vi "FYP_VI_MIDI_KeyScanDataConvert.vi"(1 "KeyScan":i16) -> (0 "MIDI Note Number":i16)   [LabVIEW 2013]
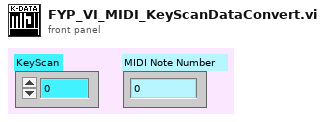
[diagram p1: front panel]
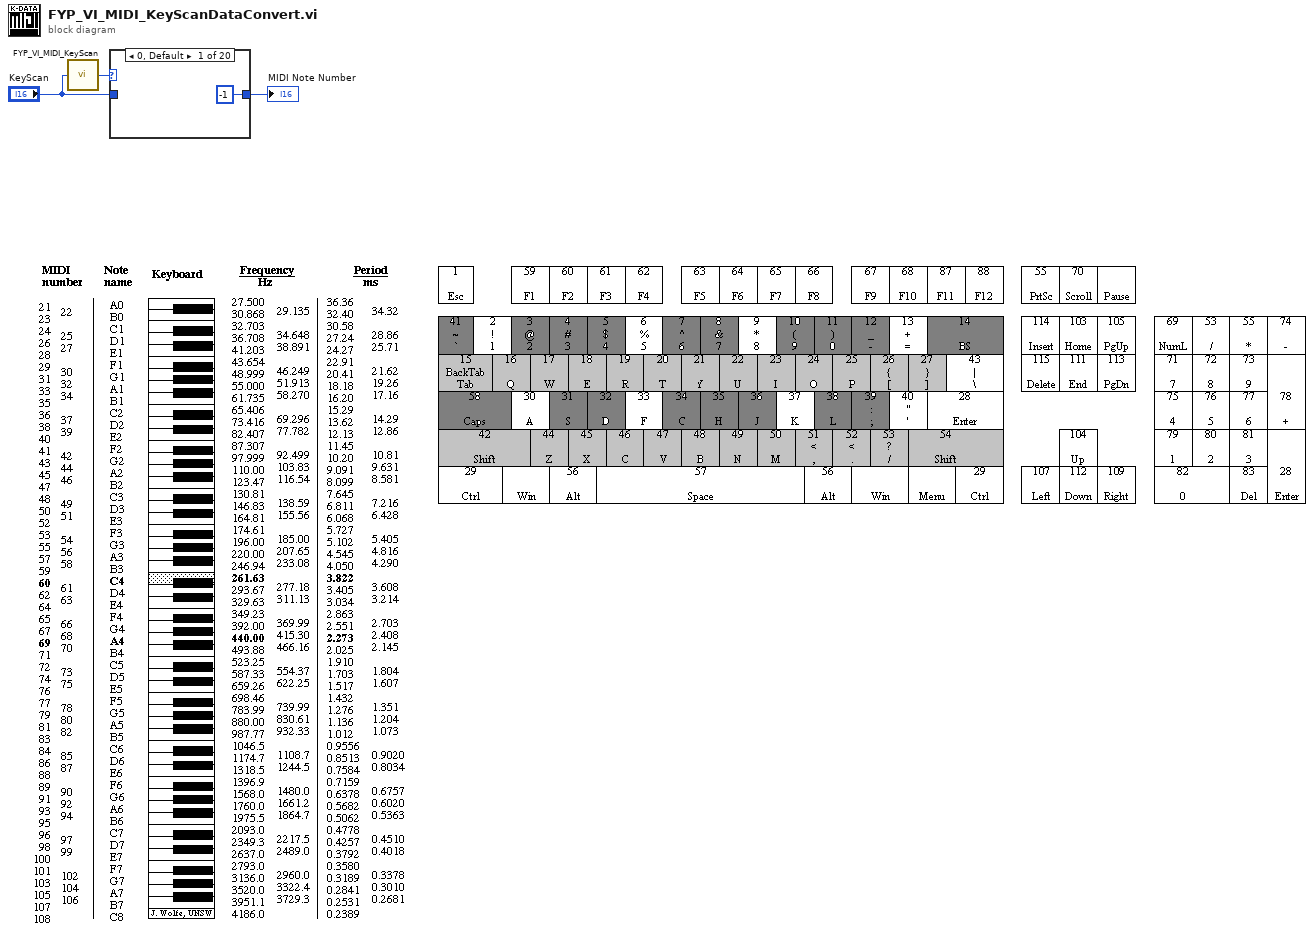
[diagram p0: block diagram]
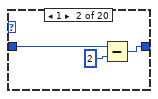
[diagram p2: hidden frame]
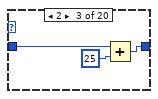
[diagram p3: hidden frame]
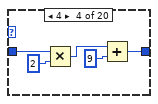
[diagram p4: hidden frame]
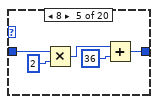
[diagram p5: hidden frame]
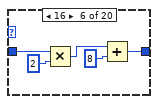
[diagram p6: hidden frame]
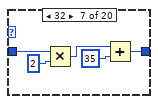
[diagram p7: hidden frame]
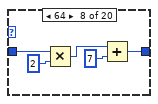
[diagram p8: hidden frame]
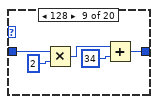
[diagram p9: hidden frame]
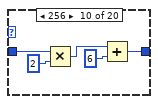
[diagram p10: hidden frame]
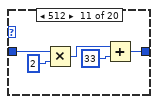
[diagram p11: hidden frame]
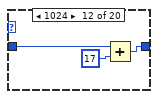
[diagram p12: hidden frame]
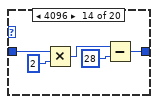
[diagram p14: hidden frame]
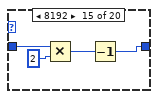
[diagram p15: hidden frame]
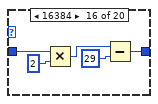
[diagram p16: hidden frame]
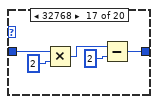
[diagram p17: hidden frame]
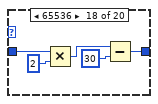
[diagram p18: hidden frame]
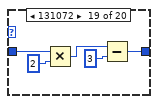
[diagram p19: hidden frame]
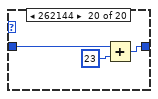
[diagram p20: hidden frame]
diagram:
  n1 = call "FYP_VI_MIDI_KeyScan.vi"("KeyScan"="KeyScan") -> ("number"=w3:u32)
  n2 = case shown="0, Default" w3 {
    tunnel: "KeyScan" -> [_ w6 w9 w15 w19 w25 w26 w32 w36 w42 w46 w51 w54 w56 w62 w65 w69 w75 w79 w85]
    tunnel: [i16 -1 ("KeyScan") w7 w10 w13 w20 w23 w27 w31 w37 w41 w47 w52 w54 w55 w60 w64 w70 w74 w80 w86] -> w1
    frame 0, Default {
    }
    frame 1 {
      n3 = Subtract(x=w6, y=i16 2) -> (x-y=w7:i16)
    }
    frame 2 {
      n4 = Add(x=w9, y=i16 25) -> (x+y=w10:i16)
    }
    frame 4 {
      n5 = Multiply(x=w15, y=i16 2) -> (x*y=w12:i16)
      n6 = Add(x=w12, y=i16 9) -> (x+y=w13:i16)
    }
    frame 8 {
      n7 = Multiply(x=w19, y=i16 2) -> (x*y=w18:i16)
      n8 = Add(x=w18, y=i16 36) -> (x+y=w20:i16)
    }
    frame 16 {
      n9 = Multiply(x=w25, y=i16 2) -> (x*y=w24:i16)
      n10 = Add(x=w24, y=i16 8) -> (x+y=w23:i16)
    }
    frame 32 {
      n11 = Multiply(x=w26, y=i16 2) -> (x*y=w30:i16)
      n12 = Add(x=w30, y=i16 35) -> (x+y=w27:i16)
    }
    frame 64 {
      n13 = Multiply(x=w32, y=i16 2) -> (x*y=w35:i16)
      n14 = Add(x=w35, y=i16 7) -> (x+y=w31:i16)
    }
    frame 128 {
      n15 = Multiply(x=w36, y=i16 2) -> (x*y=w40:i16)
      n16 = Add(x=w40, y=i16 34) -> (x+y=w37:i16)
    }
    frame 256 {
      n17 = Multiply(x=w42, y=i16 2) -> (x*y=w45:i16)
      n18 = Add(x=w45, y=i16 6) -> (x+y=w41:i16)
    }
    frame 512 {
      n19 = Multiply(x=w46, y=i16 2) -> (x*y=w50:i16)
      n20 = Add(x=w50, y=i16 33) -> (x+y=w47:i16)
    }
    frame 1024 {
      n21 = Add(x=w51, y=i16 17) -> (x+y=w52:i16)
    }
    frame 2048 {
    }
    frame 4096 {
      n22 = Multiply(x=w56, y=i16 2) -> (x*y=w59:i16)
      n23 = Subtract(x=w59, y=i16 28) -> (x-y=w55:i16)
    }
    frame 8192 {
      n24 = Multiply(x=w62, y=i16 2) -> (x*y=w61:i16)
      n25 = Decrement(x=w61) -> (x-1=w60:i16)
    }
    frame 16384 {
      n26 = Multiply(x=w65, y=i16 2) -> (x*y=w68:i16)
      n27 = Subtract(x=w68, y=i16 29) -> (x-y=w64:i16)
    }
    frame 32768 {
      n28 = Multiply(x=w69, y=i16 2) -> (x*y=w73:i16)
      n29 = Subtract(x=w73, y=i16 2) -> (x-y=w70:i16)
    }
    frame 65536 {
      n30 = Multiply(x=w75, y=i16 2) -> (x*y=w78:i16)
      n31 = Subtract(x=w78, y=i16 30) -> (x-y=w74:i16)
    }
    frame 131072 {
      n32 = Multiply(x=w79, y=i16 2) -> (x*y=w83:i16)
      n33 = Subtract(x=w83, y=i16 3) -> (x-y=w80:i16)
    }
    frame 262144 {
      n34 = Add(x=w85, y=i16 23) -> (x+y=w86:i16)
    }
  }
  "MIDI Note Number" <- w1
